vi "VFH Compute Config Space Range.vi"(1 "dA (radians)":dbl, 2 "obstacle clearance (distance)":dbl, 3 "sensor range (distance)":dbl) -> (0 "config space range (distance)":dbl)   [LabVIEW 2017, in "NI_Robotics_Vector Field Histogram.lvlib"]
uses:
  <vilib>/robotics/Obstacle Avoidance/Advanced Vector Field Histogram/NI_Robotics_Vector Field Histogram.lvlib
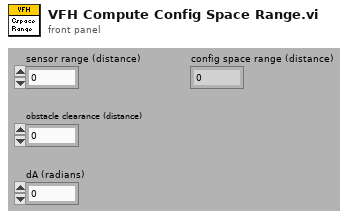
[diagram p1: front panel]
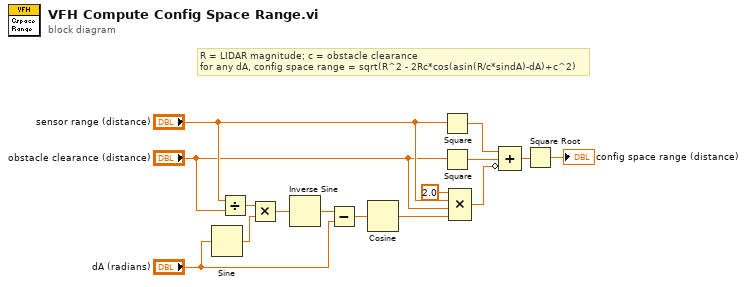
[diagram p0: block diagram]
diagram:
  # "R = LIDAR magnitude; c = obstacle clearance\nfor any dA, config space range = sqrt(R^2 - 2Rc*cos(asin(R/c*sindA)-dA)+c^2)"
  n1 = Sine(x="dA (radians)") -> (sin(x)=w14:dbl)
  n2 = Divide(x="sensor range (distance)", y="obstacle clearance (distance)") -> (x/y=w15:dbl)
  n3 = Multiply(x=w15, y=w14) -> (x*y=w13:dbl)
  n4 = Inverse Sine(1:w13) -> (0:w12:dbl)
  n5 = Subtract(x=w12, y="dA (radians)") -> (x-y=w10:dbl)
  n6 = Cosine(x=w10) -> (cos(x)=w9:dbl)
  n7 = Square(x="sensor range (distance)") -> (x^2=w5:dbl)
  n8 = Square(x="obstacle clearance (distance)") -> (x^2=w4:dbl)
  n9 = Compound Arithmetic op=MULTIPLY(2.0 ("value"), "sensor range (distance)", "obstacle clearance (distance)", w9) -> (w3:dbl)
  n10 = Compound Arithmetic op=ADD(w5, w4, invert w3) -> (w2:dbl)
  n11 = Square Root(x=w2) -> (sqrt(x)=→"config space range (distance)":dbl)
